vi "Update RD Write MSG\u0010Write write_.vi"(8 "error in (no error)":errorcluster, 10 "write?":bool, 11 "Update RD Write MSG in":refnum<class "Update RD Write MSG.lvclass">) -> (0 "error out":errorcluster, 3 "Update RD Write MSG out":refnum<class "Update RD Write MSG.lvclass">)   [LabVIEW 2014, in "Instrument Library.lvlib" / "Update RD Write MSG.lvclass"]
uses:
  Update RD Write MSG.lvclass
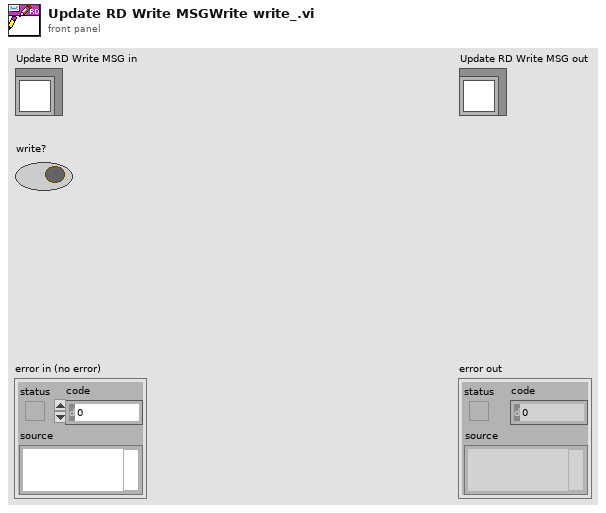
[diagram p1: front panel]
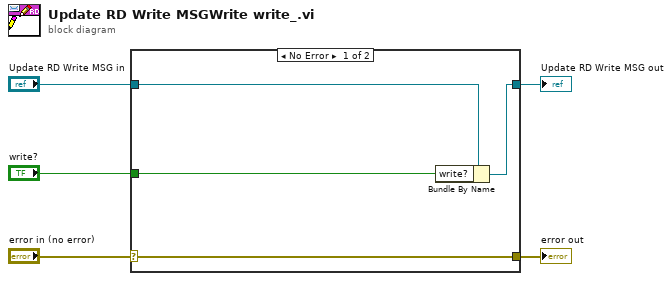
[diagram p0: block diagram]
diagram:
  n1 = case shown="No Error" "error in (no error)" {
    selector: "error in (no error)" -> [w9 w10]
    tunnel: [w9 w10] -> w4
    tunnel: [w7 w11] -> w2
    tunnel: "Update RD Write MSG in" -> [w8 w11]
    tunnel: "write?" -> [w6 _]
    frame No Error {
      n2 = Bundle By Name(cluster=w8, "write?"=w6) -> (w7:refnum<class "Update RD Write MSG.lvclass">)
    }
    frame Error {
    }
  }
  "error out" <- w4
  "Update RD Write MSG out" <- w2
